vi "Close.vi"(8 "error in (no error)":errorcluster, 11 "TCPStreamProxy in":refnum<class "TCPStream.lvclass">) -> (0 "error out":errorcluster, 3 "TCPStreamProxy out":refnum<class "TCPStream.lvclass">)   [LabVIEW 2020, in "HTTP Utils.lvlib" / "TCPStream.lvclass"]
uses:
  TCPStream.lvclass
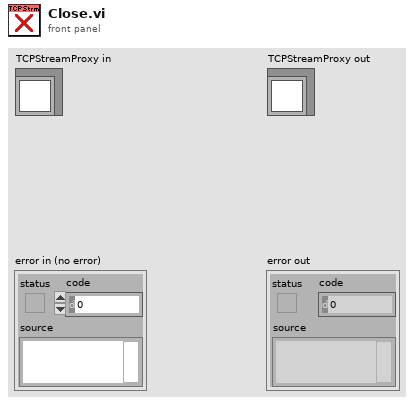
[diagram p1: front panel]
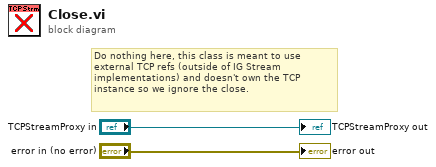
[diagram p0: block diagram]
diagram:
  # "Do nothing here, this class is meant to use external TCP refs (outside of IG Stream implementations) and doesn't own the TCP instance so we ignore the close."
  "error out" <- "error in (no error)"
  "TCPStreamProxy out" <- "TCPStreamProxy in"
